vi "Robotics Environment Simulator.vi"() -> ()   [LabVIEW 2013]
doc: "This VI starts and stops the environment simulator and serves as the master VI for your simulation code. Open and run this VI to display the environment simulator, or open the block diagram to view or modify simulation code."
uses:
  SubVIs/Behavior/Walker Mode.ctl
  <vilib>/robotics/Simulator/Engine/ctl/Step Mode.ctl
  <vilib>/Utility/miscctls.llb/LVRGBAColorTypeDef.ctl
  SubVIs/Trajectory Drawer/Trajectory Drawer.lvclass
  SubVIs/Simu Delta Robot/Simu Delta Robot.lvclass
  Common/Delta Robot Kinematics/Delta Robot Kinematics.lvclass
  <resource>/robotics/simulator/Utility/ModelBuilder/Utilities/3DController/Public/ActionType.ctl
  <resource>/robotics/simulator/Utility/ModelBuilder/Utilities/3DController/3DController.lvclass
  Common/Locus Recorder/Locus Recorder.lvclass
  <vilib>/Analysis/baseanly.llb/A x Vector.vi
  <vilib>/Analysis/baseanly.llb/Real A x B.vi
  <vilib>/Analysis/_algsub.llb/Vector Norm.vi
  <vilib>/Analysis/_algsub.llb/Real Vector Norm.vi
  <vilib>/Analysis/baseanly.llb/Outer Product.vi
  <vilib>/Analysis/baseanly.llb/Real Outer Product.vi
  <vilib>/robotics/Kinematics/Create Lie Group Matrix.vi
  <vilib>/robotics/Simulator/Interface/Simulator References/Get 3D Visual Scene Reference.vi
  <vilib>/Motion/Express/_s/nimc.ex.clearFaults.clearFaults.axis.vi
  <vilib>/Motion/Express/_s/nimc.ex.resetPosition.resetPosition.coordinate.vi
  <vilib>/Motion/Express/_s/nimc.ex.read.readExecutionData.coordinate.vi
  <vilib>/Motion/Express/_s/nimc.ex.contourMove.startContourMove.coordinate.modeFinite.vi
  <vilib>/Analysis/baseanly.llb/Real Inverse Matrix.vi
  <vilib>/Analysis/7linalg.llb/Create Special Matrix.vi
  <vilib>/Analysis/7linalg.llb/Create Special Real Matrix.vi
  <vilib>/Analysis/Matrix/Numeric/Multiply/Multiply.vi
  <vilib>/Analysis/Matrix/Numeric/Multiply/Multiply - RM,R.vi
  <vilib>/Analysis/Matrix/Numeric/Multiply/Multiply - R,RM.vi
  <vilib>/Analysis/Matrix/Numeric/Add/Add.vi
  <vilib>/Analysis/Matrix/Numeric/Add/Add - RM,RM.vi
  <vilib>/Motion/Express/_s/nimc.ex.stopMove.stop.coordinate.modeDecelerate.vi
  <vilib>/Motion/BlockNode/FB.NIMotion.xnode
  <vilib>/Motion/Express/_s/nimc.fb.contourMove.splineType.ctl
  <vilib>/robotics/Simulator/NI_Robotics_Simulator.lvlib
  <resource>/objmgr/LVODE.rc
  <vilib>/Analysis/NI_AALBase.lvlib
  <vilib>/robotics/Kinematics/NI_Kinematics.lvlib
  <vilib>/ptbypt/NI_PtbyPt.lvlib
panel:
  out "XY Graph 3":T1(graph)
  out "XY Graph 2":T1(graph)
  out "walk mode cmd":T2
  out "EF Pos Cmd":dbl[](array[numeric])
  in  "Move Robot":bool
  out "Locus Points":dbl[][](array[numeric])
  in  "walk mode":T2
  in  "Tab Control":enum32{"Page 1", "Locus Recorder"}(tab)
  in  "Generate Button":bool
  in  "Clear Button":bool
  in  "Add Button":bool
  out "Recorded Points":dbl[][](array[numeric])
  in  "speed":dbl(slide) scale=0.1..1.0
  out "p":dbl[](array[numeric])
  out "3D Picture":refnum<vi>(3d-picture)
  out "exist":bool
  out "exit":bool
  out "target pos":dbl[](array[numeric])
  out "joints":dbl[](array[numeric])
  in  "stop":bool
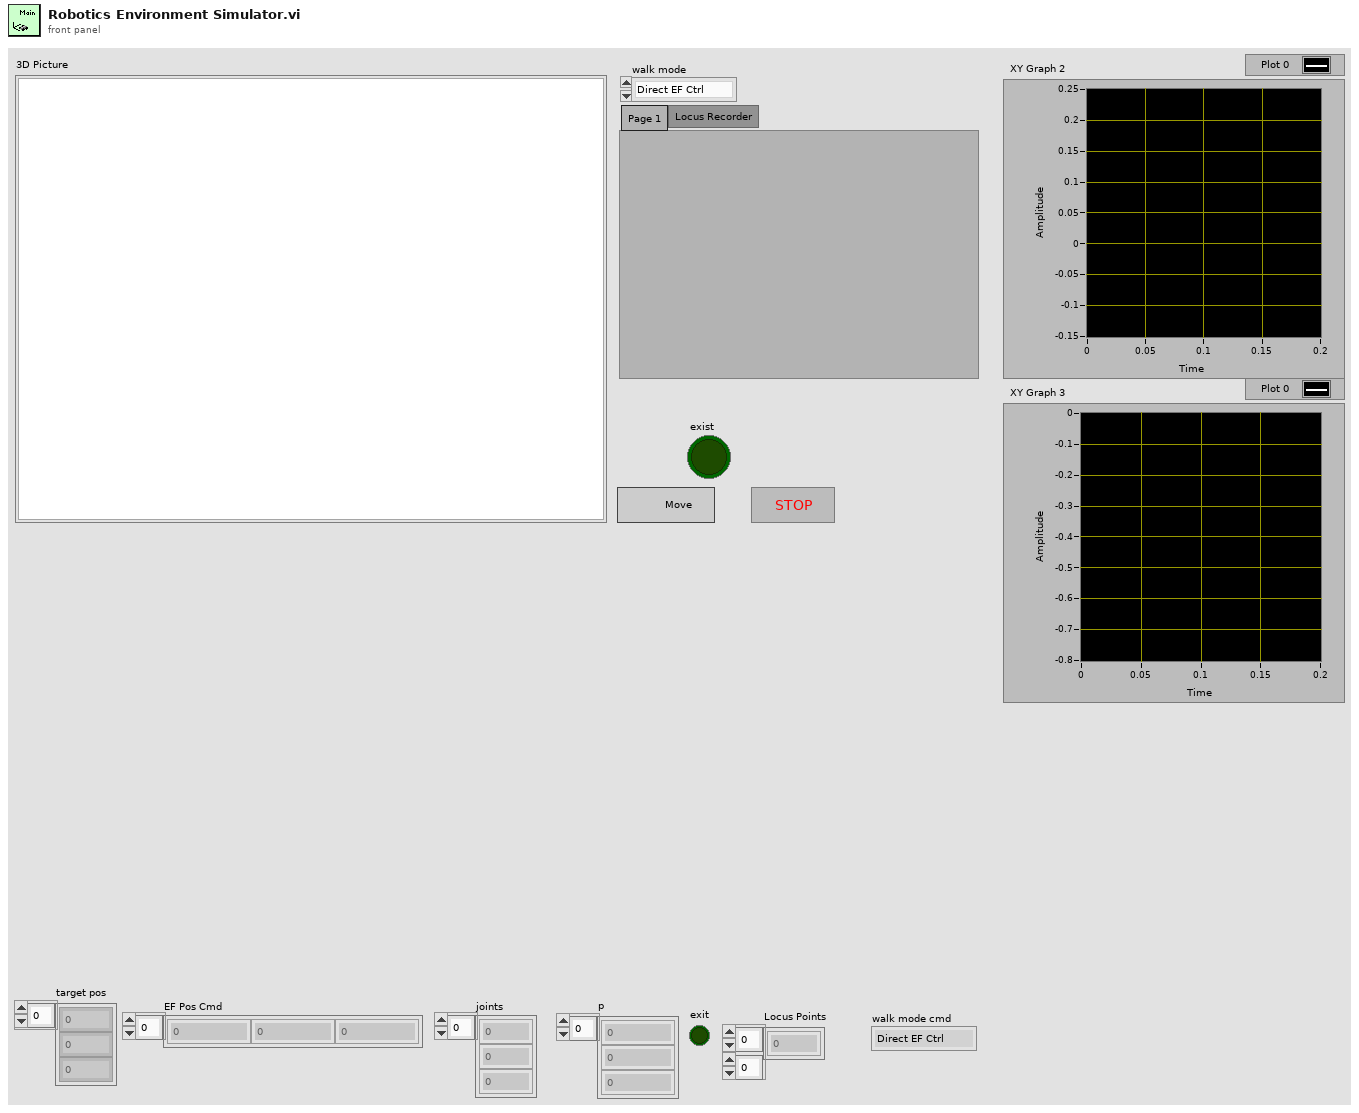
[diagram p1: front panel]
types:
  T1 = cluster{"Current Queue":dbl[], "Current Queue":dbl[]}
  T2 = typedef "Walker Mode.ctl" = enum16{"Direct EF Ctrl", "Locus Follow"}
  T3 = typedef "NI_Robotics_Simulator.lvlib/Step Mode.ctl" = u16
  T4 = typedef "LVRGBAColorTypeDef.ctl" = cluster{"Red":sgl, "Green":sgl, "Blue":sgl, "Alpha":sgl}
  T5 = typedef "NI_Robotics_Model_Builder.lvlib/3DController.lvclass/ActionType.ctl" = enum16{"None", "Trans_X", "Trans_Y", "Trans_Z", "Rot_X", "Rot_Y", "Rot_Z"}
  T6 = cluster{"Position[0]":sgl, "Position[1]":sgl, "Position[2]":sgl}
  T7 = typedef "LVPoint32TypeDef.ctl" = cluster{"Horizontal":i32, "Vertical":i32}
  T8 = typedef "LV3DPointTypeDef.ctl" = cluster{"X":sgl, "Y":sgl, "Z":sgl}
  T9 = typedef "NI_Matrix.lvlib/RealMatrix.ctl" = dbl[][]
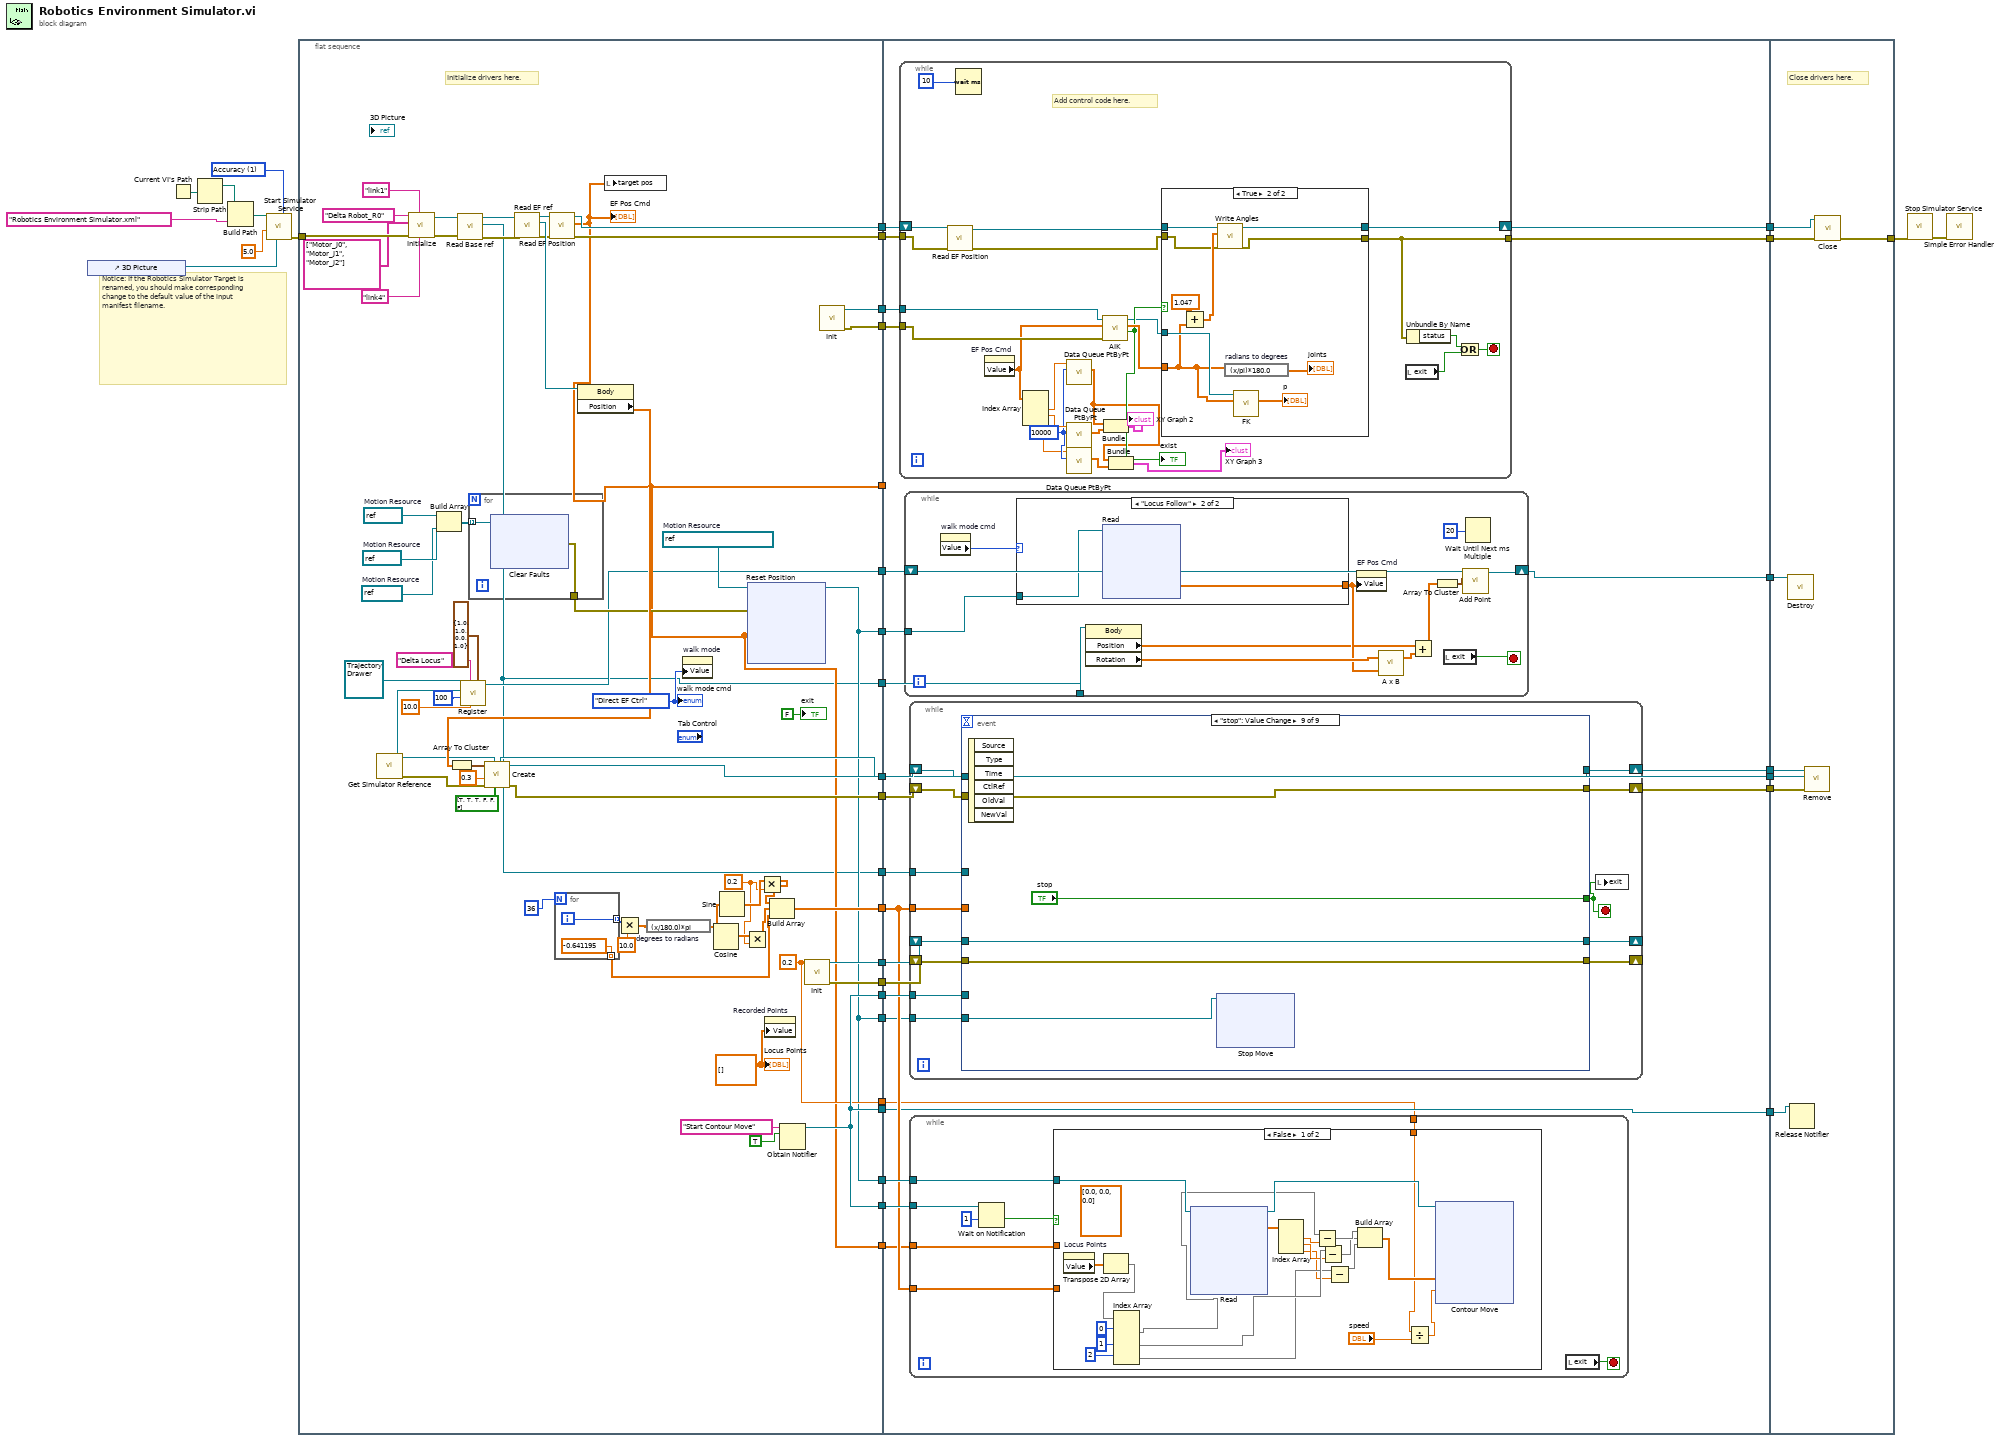
[diagram p0: block diagram]
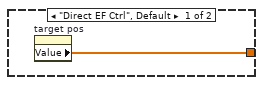
[diagram p3: hidden frame]
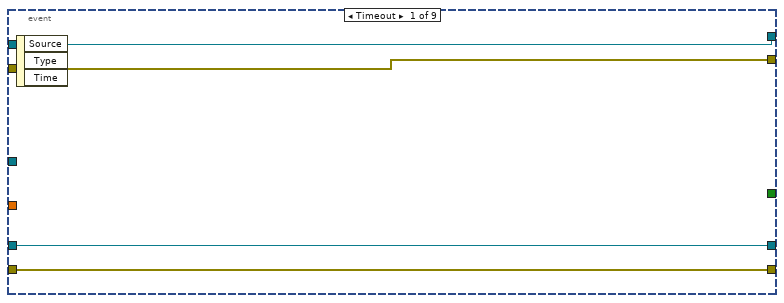
[diagram p4: hidden frame]
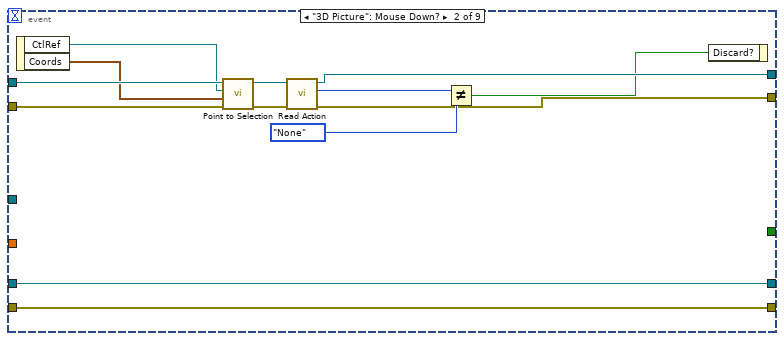
[diagram p5: hidden frame]
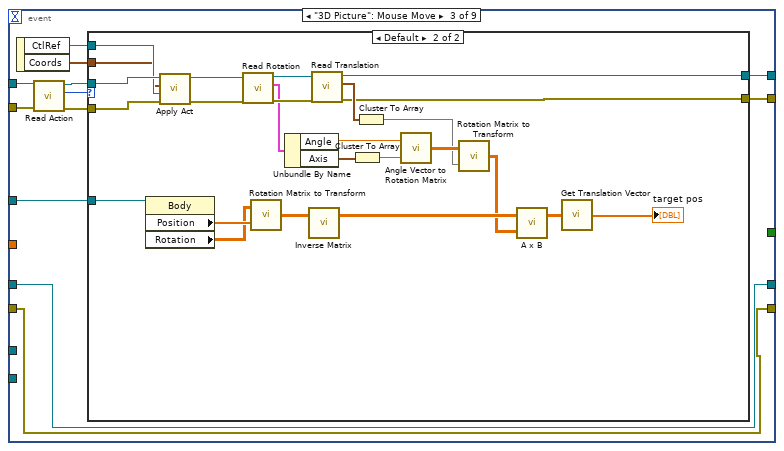
[diagram p6: hidden frame]
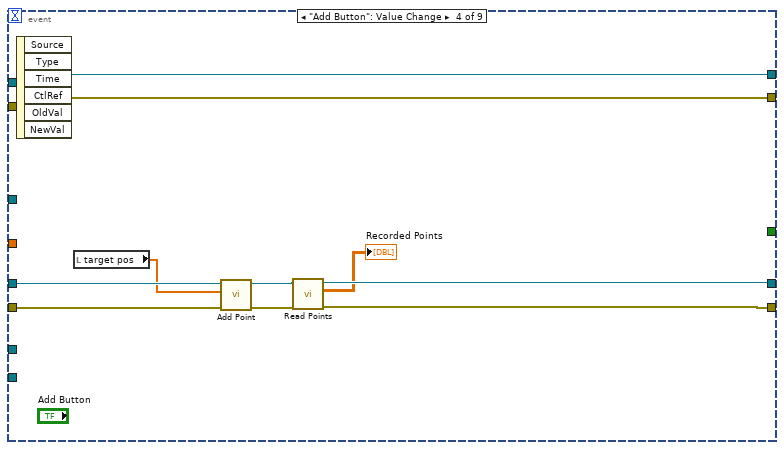
[diagram p8: hidden frame]
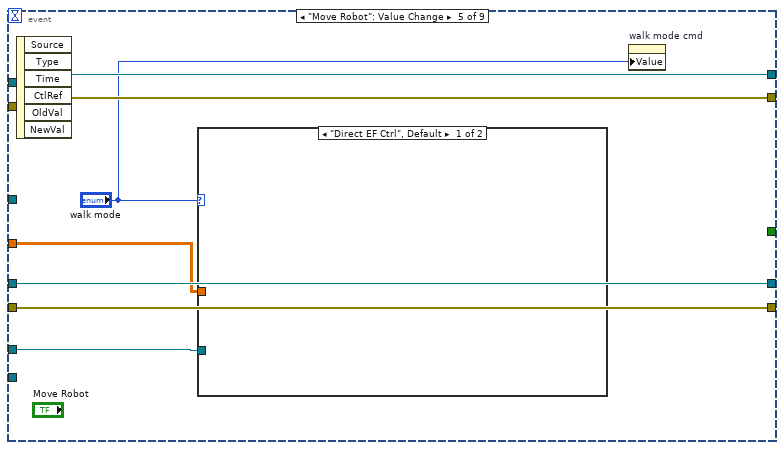
[diagram p9: hidden frame]
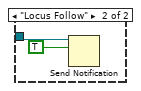
[diagram p10: hidden frame]
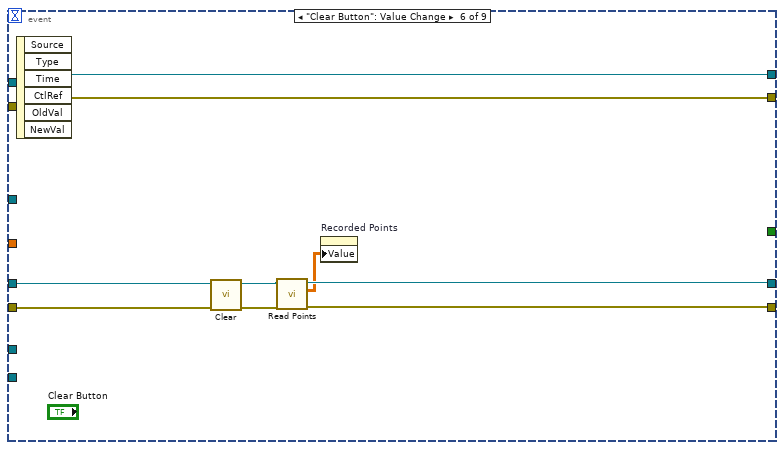
[diagram p11: hidden frame]
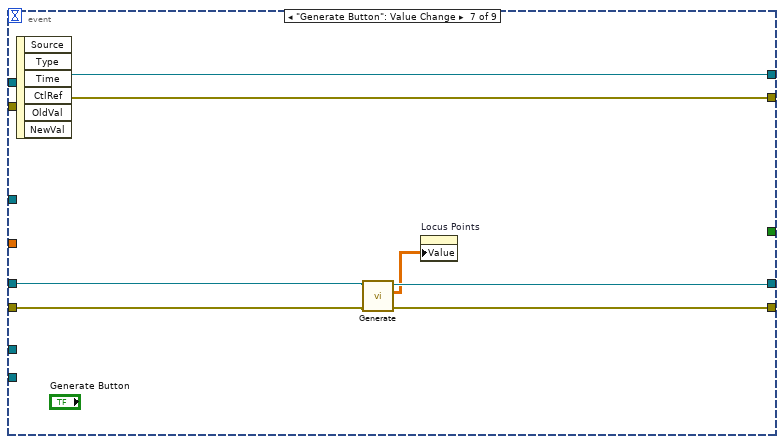
[diagram p12: hidden frame]
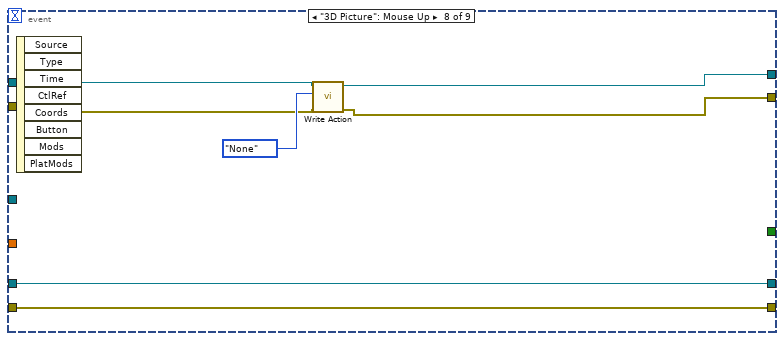
[diagram p13: hidden frame]
diagram:
  w32 = T3 1 items=["Performance", "Accuracy"] ("step mode")
  # "Notice: If the Robotics Simulator Target is renamed, you should make corresponding change to the default value of the input manifest filename."
  n1 = control-ref of="3D Picture"() -> (w24:refnum<vi>)
  n2 = Current VI's Path() -> (path=w38:path)
  n3 = Strip Path(path=w38) -> (stripped path=w37:path)  [unwired: 1 out]
  n4 = Build Path(base path=w37, name or relative path="Robotics Environment Simulator.xml" ("manifest filename")) -> (appended path=w36:path)
  n5 = call <vilib>:"Start Simulator Service.vi"("step mode"=w32, "3D picture refnum"=w24, "step size (ms)"=5.0 ("stepsize(ms)"), "manifest file"=w36) -> ("error out"=w33:errorcluster)  [unwired: 7 in]
  n6 = flat-sequence {
    tunnel: w33 -> [w92]
    tunnel: [w96] -> w31
    tunnel: [w95] -> w30
    tunnel: [w42] -> w29
    tunnel: [w93] -> w26
    tunnel: [w81] -> w23
    tunnel: [w80] -> w22
    tunnel: [w78] -> w19
    tunnel: [w77] -> w18
    tunnel: [w76] -> w16
    tunnel: [w75] -> w15
    tunnel: [w49] -> w14
    tunnel: [w65] -> w13
    tunnel: [w48] -> w12
    tunnel: [w49] -> w11
    tunnel: [w56] -> w10
    tunnel: [w56] -> w9
    tunnel: [w56] -> w7
    tunnel: [w50] -> w6
    tunnel: [w49] -> w5
    tunnel: [w48] -> w4
    tunnel: [w43] -> w3
    tunnel: [w42] -> w2
    tunnel: w31 -> [w140]
    tunnel: w30 -> [w139]
    tunnel: w29 -> [w138]
    tunnel: [w137] -> w28
    tunnel: [w136] -> w27
    tunnel: w26 -> [w135]
    tunnel: [w135] -> w25
    tunnel: w23 -> [w134]
    tunnel: w22 -> [w133]
    tunnel: [w132] -> w21
    tunnel: [w131] -> w20
    tunnel: w19 -> [w130]
    tunnel: w18 -> [w129]
    tunnel: w16 -> [w128]
    tunnel: w15 -> [w127]
    tunnel: w14 -> [w126]
    tunnel: w13 -> [w122]
    tunnel: w12 -> [_]
    tunnel: w11 -> [w125]
    tunnel: w10 -> [w124]
    tunnel: w9 -> [w123]
    tunnel: [w121] -> w8
    tunnel: w7 -> [w121]
    tunnel: w6 -> [w120]
    tunnel: w5 -> [w119]
    tunnel: w4 -> [w118]
    tunnel: w3 -> [w117]
    tunnel: w2 -> [w116]
    tunnel: [w115] -> w1
    tunnel: w28 -> [w383]
    tunnel: w27 -> [w382]
    tunnel: w25 -> [w381]
    tunnel: w21 -> [w380]
    tunnel: w20 -> [w379]
    tunnel: [w378] -> w17
    tunnel: w8 -> [w377]
    tunnel: w1 -> [w376]
    frame #0 {
      w53 = refnum<k21> "EFZ"  # Motion Resource
      w54 = refnum<k21> "EFY"  # Motion Resource
      w55 = refnum<k21> "EFX"  # Motion Resource
      w60 = 0.2
      w73 = Walker_Mode."Direct EF Ctrl" ("walk mode cmd")
      w59 = refnum<k21> "EF Coordinate Space"  # Motion Resource
      w74 = dbl[][] [] ("Locus Points")
      w50 = 0.2 ("dt")
      # "Initialize drivers here."
      n7 = call-poly <vilib>:"Get Simulator Reference.vi"() -> ("error out"=w98:errorcluster, "scene ref"=w47:refnum<vi>)  [unwired: 10 in]
      n8 = call "Initialize.vi"("EF ID"="link4" ("component ID"), "Base ID"="link1" ("component ID"), "error in (no error)"=w92, "Motor IDs"=string[] ["Motor_J0", "Motor_J1", "Motor_J2"], "Robot ID"="Delta Robot_R0" ("robot ID")) -> ("error out"=w87:errorcluster, "Simu Delta Robot"=w88:refnum<class "Simu Delta Robot.lvclass">)  [unwired: 5 in]
      n9 = Build Array(w55, w54, w53) -> (w52:refnum<k21>[])
      n10 = call-dynamic "Read Base ref.vi"("error in (no error)"=w87, "Simu Delta Robot in"=w88) -> ("error out"=w84:errorcluster, "Base ref"=w42:refnum<k20>, "Simu Delta Robot out"=w85:refnum<class "Simu Delta Robot.lvclass">)  [unwired: 7 in]
      n11 = call-dynamic "Register.vi"("Color"=T4 {"Red"=1.0, "Green"=1.0, "Blue"=0.0, "Alpha"=1.0}, "Point Size"=sgl 10.0, "Name"="Delta Locus", "Capacity"=100, "Root Sence"=w47, "Trace Drawer in"=refnum<class "Trajectory Drawer.lvclass"> refnum) -> ("Trace Drawer out"=w43:refnum<class "Trajectory Drawer.lvclass">)  [unwired: 3 in, 2 out]
      n12 = for {
        tunnel: w52 -> [w102] mode=indexing
        tunnel: [w101] -> w51
        n13 = xnode ("Clear Faults")("resource"=w102) -> ("error out"=w101:errorcluster)  [unwired: 1 in, 1 out]
      }
      n14 = call-dynamic "Read EF ref.vi"("error in (no error)"=w84, "Simu Delta Robot in"=w85) -> ("error out"=w82:errorcluster, "EF ref"=w86:refnum<k20>, "Simu Delta Robot out"=w83:refnum<class "Simu Delta Robot.lvclass">)  [unwired: 7 in]
      n15 = call-dynamic "Read EF Position.vi"("error in (no error)"=w82, "Simu Delta Robot in"=w83) -> ("error out"=w80:errorcluster, "ef pos"=w48:dbl[], "Simu Delta Robot out"=w81:refnum<class "Simu Delta Robot.lvclass">)  [unwired: 7 in]
      "EF Pos Cmd" <- w48
      n16 = for {
        N: 36 -> [_]
        tunnel: [w108] -> w70 mode=indexing
        tunnel: [-0.641195] -> w66 mode=indexing
        i -> [w108]
      }
      n17 = property class="Body"(reference=w86) -> ("Position"=w72:sgl[])  [unwired: 1 in, 2 out]
      n18 = Array To Cluster(array=w72) -> (cluster=w99:T6)
      n19 = call <resource>:"Create.vi"("Marks"=bool[] [TRUE, TRUE, TRUE, FALSE, FALSE, FALSE], "Model Root"=w47, "error in (no error)"=w98, "Scale"=0.3, "Translation"=w99) -> ("error out"=w95:errorcluster, "3DController"=w96:refnum<class "3DController.lvclass">, "Model Root out"=w93:refnum<vi>)  [unwired: 4 in]
      n20 = local write "target pos"(w48) -> ()
      n21 = Multiply(x=w70, y=10.0) -> (x*y=w68:dbl[])
      n22 = expression code="(x/180.0)*pi" "degrees to radians"(w68) -> (w67:dbl[])
      n23 = property on="walk mode" class="Enum (strict)"("Value"=w73) -> ()  [unwired: 2 in, 2 out]
      n24 = Cosine(x=w67) -> (cos(x)=w62:dbl[])
      n25 = Sine(x=w67) -> (sin(x)=w64:dbl[])
      n26 = Multiply(x=w62, y=w60) -> (x*y=w61:dbl[])
      n27 = xnode ("Reset Position")("position[]"=w48, "resource"=w59, "error in"=w51) -> ("resource out"=w49:refnum<k21>)  [unwired: 2 out]
      n28 = Multiply(x=w64, y=w60) -> (x*y=w63:dbl[])
      n29 = property on="Recorded Points" class="Arr (strict)"("Value"=w74) -> ()  [unwired: 2 in, 2 out]
      n30 = Build Array(w63, w61, w66) -> (w65:dbl[][])
      n31 = Obtain Notifier(name (unnamed)="Start Contour Move", notification data type=TRUE) -> (notifier out=w56:refnum<notifier>)  [unwired: 2 in, 2 out]
      n32 = call "Init.vi"("dt"=w50) -> ("error out"=w75:errorcluster, "Locus Recorder"=w76:refnum<class "Locus Recorder.lvclass">)  [unwired: 9 in]
      n33 = call "Init.vi"() -> ("error out"=w77:errorcluster, "Delta Robot Kin"=w78:refnum<class "Delta Robot Kinematics.lvclass">)  [unwired: 10 in]
      "exit" <- FALSE ("exit")
      "Locus Points" <- w74
      "walk mode cmd" <- w73
    }
    frame #1 {
      n34 = while {
        tunnel: w133 -> [w356]
        tunnel: [w358] -> w131
        shift-right: [w359] -> w132
        shift-left: w134 -> [w357]
        tunnel: w130 -> [w353]
        tunnel: w129 -> [w352]
        stop <- w360 stop-if-true
        w343 = 10000 ("sample length")
        # "Add control code here."
        n35 = call-dynamic "Read EF Position.vi"("error in (no error)"=w356, "Simu Delta Robot in"=w357) -> ("error out"=w354:errorcluster, "Simu Delta Robot out"=w355:refnum<class "Simu Delta Robot.lvclass">)  [unwired: 7 in, 1 out]
        n36 = Wait (ms)(milliseconds to wait=10) -> ()  [unwired: 1 out]
        n37 = property on="EF Pos Cmd" class="Arr (strict)"() -> ("Value"=w348:dbl[])  [unwired: 2 in, 2 out]
        n38 = Index Array(array=w348) -> (element #1=w347:dbl, element #2=w346:dbl, element #3=w339:dbl)  [unwired: 3 in]
        n39 = call <vilib>:"Data Queue PtByPt.vi"("sample length"=w343, "input data point"=w347) -> ("Current Queue"=w342:dbl[])  [unwired: 5 in, 4 out]
        n40 = call <vilib>:"Data Queue PtByPt.vi"("sample length"=w343, "input data point"=w346) -> ("Current Queue"=w345:dbl[])  [unwired: 5 in, 4 out]
        n41 = call <vilib>:"Data Queue PtByPt.vi"("sample length"=w343, "input data point"=w339) -> ("Current Queue"=w341:dbl[])  [unwired: 5 in, 4 out]
        n42 = call-dynamic "AIK.vi"("error in (no error)"=w352, "p"=w348, "Delta Robot Kinematics in"=w353) -> ("exist"=w350:bool, "joints"=w351:dbl[], "Delta Robot Kinematics out"=w349:refnum<class "Delta Robot Kinematics.lvclass">)  [unwired: 5 in, 1 out]
        "exist" <- w350
        n43 = Bundle("Current Queue"=w342, "Current Queue"=w345) -> (→"XY Graph 2":T1)  [unwired: 1 in]
        n44 = Bundle("Current Queue"=w342, "Current Queue"=w341) -> (→"XY Graph 3":T1)  [unwired: 1 in]
        n45 = case shown="True" w350 {
          tunnel: w351 -> [_ w367]
          tunnel: w355 -> [w365 w373]
          tunnel: w354 -> [w364 w371]
          tunnel: [w365 w370] -> w359
          tunnel: [w364 w369] -> w358
          tunnel: w349 -> [_ w368]
          frame False {
          }
          frame True {
            n46 = Add(x=1.047, y=w367) -> (x+y=w372:dbl[])
            n47 = call-dynamic "Write Angles.vi"("error in (no error)"=w371, "angles (rad)"=w372, "Simu Delta Robot in"=w373) -> ("error out"=w369:errorcluster, "Simu Delta Robot out"=w370:refnum<class "Simu Delta Robot.lvclass">)  [unwired: 7 in]
            n48 = expression code="(x/pi)*180.0" "radians to degrees"(w367) -> (→"joints":dbl[])
            n49 = call-dynamic "FK.vi"("joints"=w367, "Delta Robot Kinematics in"=w368) -> ("p"=→"p":dbl[])  [unwired: 6 in, 3 out]
          }
        }
        n50 = local read "exit"() -> (w361:bool)
        n51 = Unbundle By Name(w358) -> ("status"=w363:bool)
        n52 = Or(x=w363, y=w361) -> (x .or. y?=w360:bool)
      }
      n53 = while {
        tunnel: w126 -> [w201]
        shift-right: [w190] -> w115
        shift-left: w117 -> [w198]
        tunnel: w116 -> [w197]
        stop <- w199 stop-if-true
        n54 = property on="walk mode cmd" class="Enum (strict)"() -> ("Value"=w202:T2)  [unwired: 2 in, 2 out]
        n55 = case shown="\"Locus Follow\"" w202 {
          tunnel: w201 -> [_ w205]
          tunnel: [w203 w204] -> w195
          frame "Direct EF Ctrl", Default {
            n56 = property on="target pos" class="Arr (strict)"() -> ("Value"=w203:dbl[])  [unwired: 2 in, 2 out]
          }
          frame "Locus Follow" {
            n57 = xnode ("Read")("resource"=w205) -> ("position[] out"=w204:dbl[])  [unwired: 2 in, 4 out]
          }
        }
        n58 = property class="Body"(reference=w197) -> ("Position"=w193:sgl[], "Rotation"=w196:sgl[][])  [unwired: 1 in, 2 out]
        n59 = property on="EF Pos Cmd" class="Arr (strict)"("Value"=w195) -> ()  [unwired: 2 in, 2 out]
        n60 = call-poly <vilib>:"A x B.vi"("Vector"=w195, "A"=w196) -> ("A x Vector"=w194:dbl[])  [unwired: 1 out]
        n61 = Add(x=w193, y=w194) -> (x+y=w192:dbl[])
        n62 = Array To Cluster(array=w192) -> (cluster=w191:cluster{"[0]":dbl, "[1]":dbl, "[2]":dbl})
        n63 = local read "exit"() -> (w199:bool)
        n64 = call-dynamic "Add Point.vi"("3D Point"=w191, "Trajectory Drawer in"=w198) -> ("Trajectory Drawer out"=w190:refnum<class "Trajectory Drawer.lvclass">)  [unwired: 8 in, 1 out]
        n65 = Wait Until Next ms Multiple(millisecond multiple=u32 20) -> ()  [unwired: 1 out]
      }
      n66 = while {
        shift-right: [w224] -> w136
        shift-left: w140 -> [w226]
        shift-right: [w223] -> w137
        shift-left: w139 -> [w225]
        tunnel: w138 -> [w222]
        shift-right: [w218] -> _
        shift-left: w128 -> [w220]
        shift-right: [w217] -> _
        shift-left: w127 -> [w219]
        tunnel: w122 -> [w216]
        tunnel: w124 -> [w215]
        tunnel: w119 -> [w214]
        stop <- w221 stop-if-true
        n67 = event shown="[8] \"stop\": Value Change" {
          selector: _ -> [_ _ _ _ _ _ _ _ _]
          dyn-events: _ -> [_ _ _ _ _ _ _ _ _]
          timeout: _ -> [_ _ _ _ _ _ _ _ _]
          tunnel: w226 -> [w230 w239 w255 w292 w299 w310 w317 w323 w330]
          tunnel: w225 -> [w229 w238 w254 w291 w298 w309 w316 w322 w329]
          tunnel: [w230 w235 w247 w292 w299 w310 w317 w321 w330] -> w224
          tunnel: [w229 w234 w246 w291 w298 w309 w316 w320 w329] -> w223
          tunnel: w222 -> [_ _ w248 _ _ _ _ _ _]
          tunnel: [_ _ _ _ _ _ _ _ "stop"] -> w221
          tunnel: w220 -> [w228 w232 w245 w290 w297 w308 w315 w319 w327]
          tunnel: w219 -> [w227 w231 w244 w288 w296 w307 w314 w318 w326]
          tunnel: [w228 w232 w245 w284 w297 w305 w313 w319 w327] -> w218
          tunnel: [w227 w231 w244 w285 w296 w303 w312 w318 w326] -> w217
          tunnel: w216 -> [_ _ _ _ w294 _ _ _ _]
          tunnel: w215 -> [_ _ _ _ w293 _ _ _ _]
          tunnel: w214 -> [_ _ _ _ _ _ _ _ w325]
          event Timeout {
            n68 = event-data() -> ()  [unwired: 1 in, 3 out]
          }
          event "3D Picture": Mouse Down? {
            n69 = event-data() -> ("CtlRef"=w237:refnum<vi>, "Coords"=w236:T7)  [unwired: 1 in]
            n70 = call-dynamic "Point to Selection.vi"("error in (no error)"=w238, "Coords"=w236, "CtlRef"=w237, "3DController in"=w239) -> ("error out"=w243:errorcluster, "3DController out"=w242:refnum<class "3DController.lvclass">)  [unwired: 6 in]
            n71 = call-dynamic "Read Action.vi"("error in (no error)"=w243, "3DController in"=w242) -> ("error out"=w234:errorcluster, "Action"=w241:T5, "3DController out"=w235:refnum<class "3DController.lvclass">)  [unwired: 7 in]
            n72 = Not Equal?(x=w241, y=ActionType."None") -> (x != y?=w233:bool)
            n73 = event-data("Discard?"=w233) -> ()  [unwired: 1 in, 1 out]
          }
          event "3D Picture": Mouse Move {
            n74 = event-data() -> ("CtlRef"=w250:refnum<vi>, "Coords"=w249:T7)  [unwired: 1 in]
            n75 = call-dynamic "Read Action.vi"("error in (no error)"=w254, "3DController in"=w255) -> ("error out"=w251:errorcluster, "Action"=w253:T5, "3DController out"=w252:refnum<class "3DController.lvclass">)  [unwired: 7 in]
            n76 = case shown="Default" w253 {
              tunnel: w252 -> [w257 w266]
              tunnel: w251 -> [w256 w265]
              tunnel: w250 -> [_ w264]
              tunnel: w249 -> [_ w263]
              tunnel: w248 -> [_ w262]
              tunnel: [w257 w259] -> w247
              tunnel: [w256 w258] -> w246
              frame "None" {
              }
              frame Default {
                n77 = property class="Body"(reference=w262) -> ("Position"=w271:sgl[], "Rotation"=w270:sgl[][])  [unwired: 1 in, 2 out]
                n78 = call-dynamic "Apply Act.vi"("error in (no error)"=w265, "3D Scene"=w264, "End Point"=w263, "3DController in"=w266) -> ("error out"=w281:errorcluster, "3DController out"=w282:refnum<class "3DController.lvclass">)  [unwired: 6 in]
                n79 = call-dynamic "Read Rotation.vi"("error in (no error)"=w281, "3DController in"=w282) -> ("error out"=w279:errorcluster, "Rotation"=w278:cluster{"Axis":T8, "Angle":sgl}, "3DController out"=w280:refnum<class "3DController.lvclass">)  [unwired: 7 in]
                n80 = call <vilib>:"Rotation Matrix to Transform.vi"("translation vector"=w271, "rotation matrix"=w270) -> ("transform"=w269:T9)
                n81 = Unbundle By Name(w278) -> ("Angle"=w275:sgl, "Axis"=w277:T8)
                n82 = call-poly <vilib>:"Inverse Matrix.vi"("Input Matrix"=w269) -> ("Inverse Matrix"=w268:T9)  [unwired: 1 in, 1 out]
                n83 = call-dynamic "Read Translation.vi"("error in (no error)"=w279, "3DController in"=w280) -> ("error out"=w258:errorcluster, "3D Point"=w273:T8, "3DController out"=w259:refnum<class "3DController.lvclass">)  [unwired: 7 in]
                n84 = Cluster To Array(cluster=w277) -> (array=w276:sgl[])
                n85 = Cluster To Array(cluster=w273) -> (array=w272:sgl[])
                n86 = call <vilib>:"Angle Vector to Rotation Matrix.vi"("vector"=w276, "angle"=w275) -> ("rotation matrix"=w274:T9)
                n87 = call <vilib>:"Rotation Matrix to Transform.vi"("translation vector"=w272, "rotation matrix"=w274) -> ("transform"=w267:T9)
                n88 = call-poly <vilib>:"A x B.vi"("B"=w267, "A"=w268) -> ("A x B"=w261:T9)  [unwired: 1 out]
                n89 = call <vilib>:"Get Translation Vector.vi"("transform"=w261) -> ("translation vector"=→"target pos":dbl[])
              }
            }
          }
          event "Add Button": Value Change {
            n90 = event-data() -> ()  [unwired: 1 in, 6 out]
            n91 = local read "target pos"() -> (w289:dbl[])
            n92 = call-dynamic "Add Point.vi"("error in (no error)"=w288, "point"=w289, "Locus Recorder in"=w290) -> ("error out"=w286:errorcluster, "Locus Recorder out"=w287:refnum<class "Locus Recorder.lvclass">)  [unwired: 7 in]
            n93 = call-dynamic "Read Points.vi"("error in (no error)"=w286, "Locus Recorder in"=w287) -> ("error out"=w285:errorcluster, "Points"=→"Recorded Points":dbl[][], "Locus Recorder out"=w284:refnum<class "Locus Recorder.lvclass">)  [unwired: 7 in]
          }
          event "Move Robot": Value Change {
            n94 = event-data() -> ()  [unwired: 1 in, 6 out]
            n95 = case shown="\"Direct EF Ctrl\", Default" "walk mode" {
              tunnel: w294 -> [_ _]
              tunnel: w293 -> [_ w301]
              frame "Direct EF Ctrl", Default {
              }
              frame "Locus Follow" {
                n96 = Send Notification(notification=TRUE, notifier=w301) -> ()  [unwired: 1 in, 2 out]
              }
            }
            n97 = property on="walk mode cmd" class="Enum (strict)"("Value"="walk mode") -> ()  [unwired: 2 in, 2 out]
          }
          event "Clear Button": Value Change {
            n98 = event-data() -> ()  [unwired: 1 in, 6 out]
            n99 = call-dynamic "Clear.vi"("error in (no error)"=w307, "Locus Recorder in"=w308) -> ("error out"=w304:errorcluster, "Locus Recorder out"=w306:refnum<class "Locus Recorder.lvclass">)  [unwired: 8 in]
            n100 = call-dynamic "Read Points.vi"("error in (no error)"=w304, "Locus Recorder in"=w306) -> ("error out"=w303:errorcluster, "Points"=w302:dbl[][], "Locus Recorder out"=w305:refnum<class "Locus Recorder.lvclass">)  [unwired: 7 in]
            n101 = property on="Recorded Points" class="Arr (strict)"("Value"=w302) -> ()  [unwired: 2 in, 2 out]
          }
          event "Generate Button": Value Change {
            n102 = event-data() -> ()  [unwired: 1 in, 6 out]
            n103 = call-dynamic "Generate.vi"("error in (no error)"=w314, "Locus Recorder in"=w315) -> ("error out"=w312:errorcluster, "Points"=w311:dbl[][], "Locus Recorder out"=w313:refnum<class "Locus Recorder.lvclass">)  [unwired: 7 in]
            n104 = property on="Locus Points" class="Arr (strict)"("Value"=w311) -> ()  [unwired: 2 in, 2 out]
          }
          event "3D Picture": Mouse Up {
            n105 = event-data() -> ()  [unwired: 1 in, 8 out]
            n106 = call-dynamic "Write Action.vi"("error in (no error)"=w322, "Action"=ActionType."None", "3DController in"=w323) -> ("error out"=w320:errorcluster, "3DController out"=w321:refnum<class "3DController.lvclass">)  [unwired: 7 in]
          }
          event "stop": Value Change {
            n107 = event-data() -> ()  [unwired: 1 in, 6 out]
            n108 = xnode ("Stop Move")("resource"=w325) -> ()  [unwired: 2 in, 3 out]
          }
        }
        n109 = local write "exit"(w221) -> ()
      }
      n110 = while {
        tunnel: w125 -> [w148]
        tunnel: w123 -> [w147]
        tunnel: w122 -> [w144]
        tunnel: w120 -> [w142]
        tunnel: w118 -> [w141]
        stop <- w143 stop-if-true
        n111 = Wait on Notification(notifier=w147, timeout in ms (-1)=1) -> (timed out?=w145:bool)  [unwired: 2 in, 3 out]
        n112 = case shown="False" w145 {
          tunnel: w148 -> [w169 _]
          tunnel: w144 -> [_ _]
          tunnel: w142 -> [w150 _]
          tunnel: w141 -> [_ _]
          frame False {
            (unwired) dbl[] [0.0, 0.0, 0.0]
            n113 = property on="Locus Points" class="Arr (strict)"() -> ("Value"=w160:dbl[][])  [unwired: 2 in, 2 out]
            n114 = Transpose 2D Array(2D array=w160) -> (transposed array=w159:dbl[][])
            n115 = Index Array(array=w159, index (row) #1=0 ("index (row)"), index (row) #2=1 ("index (row)"), index (row) #3=2 ("index (row)")) -> (element #1=w164:dbl[], element #2=w163:dbl[], element #3=w162:dbl[])  [unwired: 3 in]
            n116 = xnode ("Read")("resource"=w169) -> ("position[] out"=w158:dbl[], "resource out"=w166:refnum<k21>)  [unwired: 2 in, 3 out]
            n117 = Index Array(array=w158) -> (element #1=w157:dbl, element #2=w156:dbl, element #3=w155:dbl)  [unwired: 3 in]
            n118 = Subtract(x=w164, y=w157) -> (x-y=w154:dbl[])
            n119 = Subtract(x=w163, y=w156) -> (x-y=w153:dbl[])
            n120 = Subtract(x=w162, y=w155) -> (x-y=w152:dbl[])
            n121 = Build Array(w154, w153, w152) -> (w161:dbl[][])
            n122 = Divide(x=w150, y="speed") -> (x/y=w149:dbl)
            n123 = xnode ("Contour Move")("points[][]"=w161, "interval"=w149, "resource"=w166) -> ()  [unwired: 4 in, 3 out]
          }
          frame True {
          }
        }
        n124 = local read "exit"() -> (w143:bool)
      }
    }
    frame #2 {
      # "Close drivers here."
      n125 = call-dynamic "Destroy.vi"("Trajectory Drawer in"=w376) -> ()  [unwired: 8 in, 3 out]
      n126 = Release Notifier(notifier=w377) -> ()  [unwired: 2 in, 3 out]
      n127 = call-dynamic "Remove.vi"("error in (no error)"=w383, "Model Root"=w381, "3DController in"=w382) -> ()  [unwired: 7 in, 2 out]
      n128 = call-dynamic "Close.vi"("error in (no error)"=w379, "Simu Delta Robot in"=w380) -> ("error out"=w378:errorcluster)  [unwired: 8 in, 1 out]
    }
  }
  n129 = call <vilib>:"Stop Simulator Service.vi"("error in (no error)"=w17) -> ("error out"=w34:errorcluster)  [unwired: 10 in]
  n130 = call <vilib>:"Simple Error Handler.vi"("error in (no error)"=w34) -> ()  [unwired: 4 in, 5 out]
